vi "Write Menu Items.vi"(8 "error in (no error)":errorcluster, 10 "Menu Items":T1, 11 "Front Panel Menu in":refnum<class "Front Panel Menu.lvclass">) -> (0 "error out":errorcluster, 3 "Front Panel Menu out":refnum<class "Front Panel Menu.lvclass">)   [LabVIEW 2024, in "Front Panel Menu.lvclass"]
uses:
  Front Panel Menu.lvclass
  Type Def/Menu Item Group.ctl
  Type Def/Menu Item.ctl
  Front Panel Menu.lvclass/Front Panel Menu.ctl
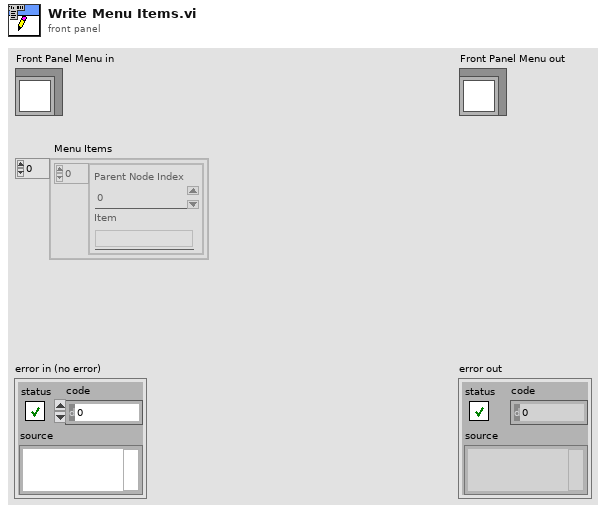
[diagram p1: front panel]
types:
  T1 = typedef "Menu Item Group.ctl" = cluster{"Array":T2[]}[]
  T2 = typedef "Menu Item.ctl" = cluster{"Parent Node Index":i32, "Item":string}
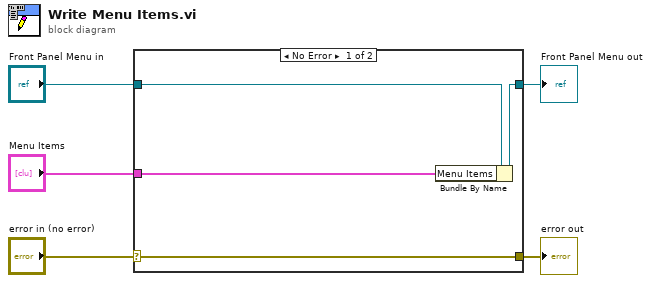
[diagram p0: block diagram]
diagram:
  n1 = case shown="No Error" "error in (no error)" {
    selector: "error in (no error)" -> [w9 w10]
    tunnel: [w9 w10] -> w4
    tunnel: [w7 w11] -> w2
    tunnel: "Front Panel Menu in" -> [w8 w11]
    tunnel: "Menu Items" -> [w6 _]
    frame No Error {
      n2 = Bundle By Name(cluster=w8, "Menu Items"=w6) -> (w7:refnum<class "Front Panel Menu.lvclass">)
    }
    frame Error {
    }
  }
  "error out" <- w4
  "Front Panel Menu out" <- w2
